vi "UnitTest-FileOrDirCreated.vi"(8 "error in":errorcluster) -> (0 "error out":errorcluster)   [LabVIEW 2014]
uses:
  TableLogger_Actor/TableLoggerConfig.ctl
  TableLogger_Actor/TableLoggerTypes.ctl
  TableLogger_Actor/TableLoggerBackupConfig.ctl
  <vilib>/ActorFramework/Message Enqueuer/Message Enqueuer.lvclass/Message Enqueuer.ctl
  <vilib>/ActorFramework/Message Enqueuer/Enqueue.vi
  <vilib>/ActorFramework/Message Priority Queue/Priority Enqueue.vi
  <vilib>/ActorFramework/Stop Msg/Stop Msg.lvclass
  <vilib>/addons/_JKI Toolkits/Caraya/classes/Assert/Assert.lvclass
  TableLogger_Actor/TableLogger_Actor/TableLogger_Actor.lvclass
  <vilib>/addons/_JKI Toolkits/Caraya/classes/Test/Test.lvclass
  TableLogger_Actor/TableLogger_Actor.lvlib
panel:
  # "Connector Pane"
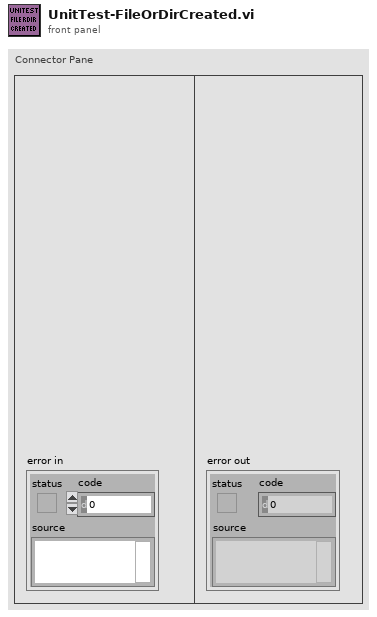
[diagram p1: front panel]
types:
  T1 = typedef "TableLogger_Actor.lvlib/TableLoggerConfig.ctl" = cluster{"TableLogger":T2, "DB File Path":path, "DB Backup Config":T3}
  T2 = typedef "TableLogger_Actor.lvlib/TableLoggerTypes.ctl" = enum16{"CSV Logger", "SQLite Logger"}
  T3 = typedef "TableLogger_Actor.lvlib/TableLoggerBackupConfig.ctl" = cluster{"Directory":path, "UTC Time Format":bool, "On Launch":bool, "Interval (Hours)":dbl, "Size Multiples (Bytes)":i32}
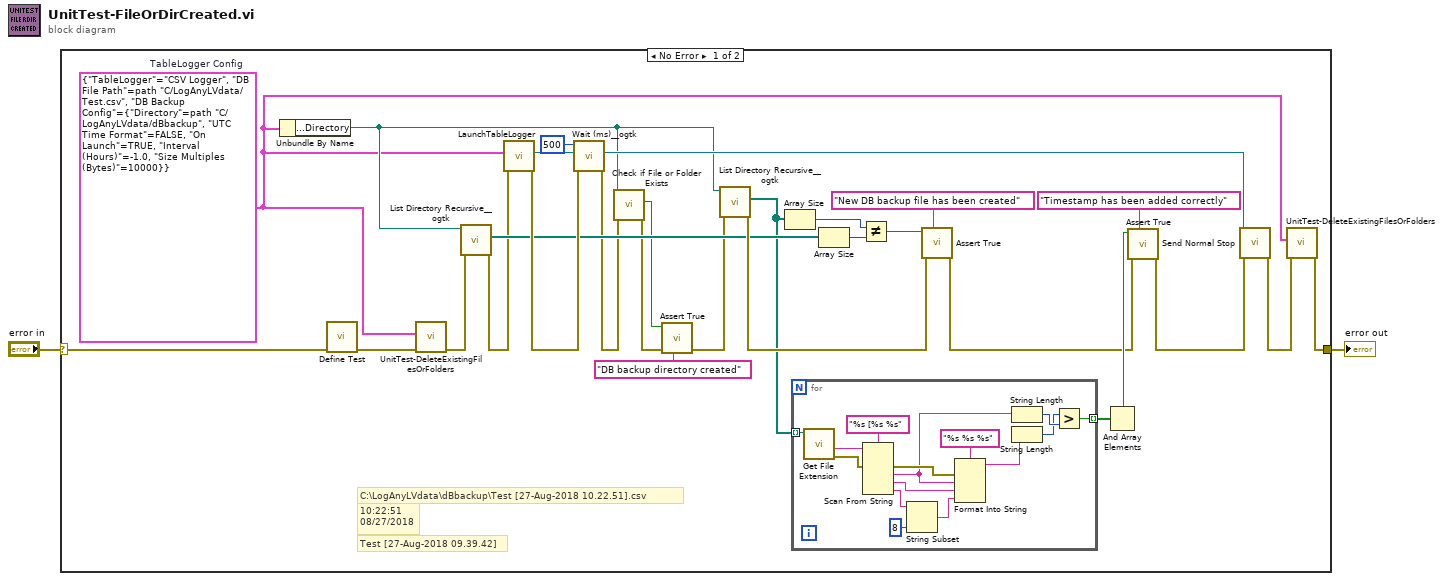
[diagram p0: block diagram]
diagram:
  n1 = case shown="No Error" "error in" {
    selector: "error in" -> [w15 w46]
    tunnel: [w9 w46] -> w1
    frame No Error {
      w5 = T1 {"TableLogger"=enum."CSV Logger", "DB File Path"=path "C:/LogAnyLVdata/Test.csv", "DB Backup Config"={"Directory"=path "C:/LogAnyLVdata/dBbackup", "UTC Time Format"=FALSE, "On Launch"=TRUE, "Interval (Hours)"=-1.0, "Size Multiples (Bytes)"=10000}}  # TableLogger Config
      # "Test [27-Aug-2018 09.39.42]"
      # "10:22:51\n08/27/2018"
      # "C:\\LogAnyLVdata\\dBbackup\\Test [27-Aug-2018 10.22.51].csv"
      n2 = Unbundle By Name(w5) -> ("DB Backup Config.Directory"=w6:path)
      n3 = call <vilib>:"Define Test.vi"("error in (no error)"=w15) -> ("error out"=w8:errorcluster)  [unwired: 10 in]
      n4 = call "UnitTest-DeleteExistingFilesOrFolders.vi"("error in (no error)"=w8, "Config IN"=w5) -> ("error out"=w7:errorcluster)  [unwired: 9 in]
      n5 = call "List Directory Recursive__ogtk.vi"("error in (no error)"=w7, "Path"=w6) -> ("error out"=w14:errorcluster, "file paths"=w26:path[])  [unwired: 6 in, 2 out]
      n6 = call "LaunchTableLogger.vi"("error in (no error)"=w14, "TableLogger Config"=w5) -> ("error out"=w30:errorcluster, "TableLogger Actor's Enqueuer"=w19:refnum<class "Message Enqueuer.lvclass">)  [unwired: 6 in, 2 out]
      n7 = call "Wait (ms)__ogtk.vi"("error in (no error)"=w30, "milliseconds to wait"=u32 500) -> ("error out"=w4:errorcluster)  [unwired: 8 in, 1 out]
      n8 = call <vilib>:"Check if File or Folder Exists.vi"("error in (no error)"=w4, "path"=w6) -> ("error out"=w3:errorcluster, "file or folder exists?"=w13:bool)  [unwired: 7 in, 1 out]
      n9 = call <vilib>:"Assert True.vi"("Label"="DB backup directory created", "error in (no error)"=w3, "True?"=w13) -> ("error out"=w11:errorcluster)  [unwired: 8 in]
      n10 = call "List Directory Recursive__ogtk.vi"("error in (no error)"=w11, "Path"=w6) -> ("error out"=w27:errorcluster, "file paths"=w25:path[])  [unwired: 6 in, 2 out]
      n11 = Array Size(array=w25) -> (size(s)=w18:i32)
      n12 = for {
        tunnel: w25 -> [w45] mode=indexing
        tunnel: [w32] -> w23 mode=indexing
        n13 = call <vilib>:"Get File Extension.vi"("file"=w45) -> ("error out"=w31:errorcluster, "filename without extension"=w39:string)  [unwired: 7 in, 2 out]
        n14 = Scan From String(format string="%s [%s %s", input string=w39, error in=w31) -> (error out=w44:errorcluster, output 1=w36:string, output 2=w37:string, output 3=w42:string)  [unwired: 4 in, 2 out]
        n15 = String Subset(string=w42, length (rest)=8 ("length (rest)")) -> (substring=w38:string)  [unwired: 1 in]
        n16 = Format Into String(format string="%s %s %s", error in=w44, w36, w37, w38) -> (resulting string=w35:string)  [unwired: 1 in, 1 out]
        n17 = String Length(string=w36) -> (length=w34:i32)
        n18 = String Length(string=w35) -> (length=w33:i32)
        n19 = Greater?(x=w33, y=w34) -> (0:w32:bool)
      }
      n20 = Array Size(array=w26) -> (size(s)=w17:i32)
      n21 = Not Equal?(x=w18, y=w17) -> (x != y?=w28:bool)
      n22 = call <vilib>:"Assert True.vi"("Label"="New DB backup file has been created", "error in (no error)"=w27, "True?"=w28) -> ("error out"=w21:errorcluster)  [unwired: 8 in]
      n23 = And Array Elements(Boolean array=w23) -> (logical AND=w22:bool)
      n24 = call <vilib>:"Assert True.vi"("Label"="Timestamp has been added correctly", "error in (no error)"=w21, "True?"=w22) -> ("error out"=w20:errorcluster)  [unwired: 8 in]
      n25 = call <vilib>:"Send Normal Stop.vi"("error in (no error)"=w20, "Message Enqueuer"=w19) -> ("error out"=w10:errorcluster)  [unwired: 9 in]
      n26 = call "UnitTest-DeleteExistingFilesOrFolders.vi"("error in (no error)"=w10, "Config IN"=w5) -> ("error out"=w9:errorcluster)  [unwired: 9 in]
    }
    frame Error {
    }
  }
  "error out" <- w1
